vi "TCP server 一对多通讯.vi"() -> ()   [LabVIEW 2015]
uses:
  <vilib>/Analysis/NI_AALBase.lvlib
panel:
  in  "port":u16
  in  "stop":bool
  out "Waveform Graph":dbl[](graph)=[0.0, -0.3446629861261414, 0.6449819459130841, -0.866106479495641, 0.9838729732815561, -0.9870668288033351, 0.878021082565634, -0.6716184455574631, 0.3929433336250866, -0.07396159032953767, -0.25032118712159324, 0.5457579020007043, -0.7825896428232234, 0.9382637669810894, -0.9993074889815294, 0.9621466451128676, -0.8328794880822399, 0.6261206676264622, -0.36311182915767126, 0.0693472019188715, 0.22801633623988113, -0.5027030305125276, 0.7315863059803936, -0.8965016644442846, 0.9854858291916155, -0.9933879258623504, 0.9218598941944436, -0.7787864999433254, 0.5772565526765175, -0.33420418461912077, 0.06886184239247578, 0.1988341088361352, -0.4497566031034409, 0.6669125839906785, -0.83649898302553, 0.9486396514480464, -0.9977828240105574, 0.9827661921181812, -0.9065799590979673, 0.7758761586666735, -0.6002844704019976, 0.3916007514616761, -0.16291497204376829, -0.07225901034618203, 0.30079735532851715, -0.5106798662431301, 0.6915713530529537, -0.8352511156797895, 0.9358828015976429, -0.9901275470744442, 0.997112242978794, -0.9582716672425805, 0.8770879789061665, -0.7587537174921901, 0.6097851702353462, -0.43761202654463116, 0.25016696100073327, -0.055495526672846324, -0.1385971483755034, 0.3248505585398878, -0.49679581216189184, 0.6489412953319964, -0.7768964578302177, 0.8774362101337545, -0.9485108543705275, 0.9892082753602621, -0.9996763045465049, 0.9810137849159348, -0.9351389766759363, 0.8646436335742596, -0.7726404372844417, 0.6626105919055042, -0.5382573376516607, 0.40337001948772405, -0.26170220948298023, 0.11686628573757678, 0.027754141792931248, -0.16907346713967436, 0.3043552605745123, -0.4312462762906236, 0.5477946760053648, -0.6524541934721085, 0.7440761832213633, -0.8218916033501608, 0.8854849932658432, -0.9347624402955282, 0.9699154012496086, -0.9913820727887072, 0.9998078027986025, -0.9960058171624511, 0.9809193135871277, -0.9555857556896089, 0.9211039935631101, -0.878604646809285, 0.8292240161144818, -0.7740816419367104, 0.7142615045606484, -0.6507967584456191, 0.5846578144089939, -0.5167435241375766, 0.4478751807836437, -0.3787930247242358, 0.31015493258496235, -0.24253696800529956, 0.17643548209795307, -0.112270468033949, 0.05038989577020649, 0.008925222046267417, -0.06545525495299609, 0.11903606448288666, -0.16955296546409745, 0.21693467872241692, -0.26114739000849074, 0.30218900684481415, -0.3400836840953238, 0.3748766705541803, -0.40662951278131604, 0.4354156387531364, -0.461316332559608, 0.4844171022317741, -0.5048044356639747, 0.522562934321303, -0.5377728108040681, 0.5505077341839772, -0.5608330061412039, 0.568804051134239, -0.5744652049513441, 0.5778487878598408]
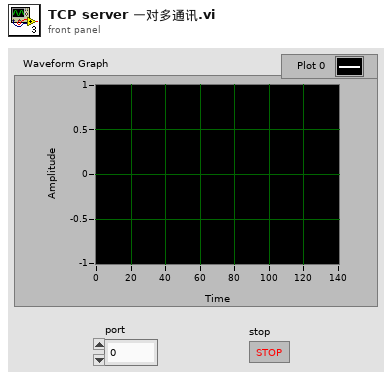
[diagram p1: front panel]
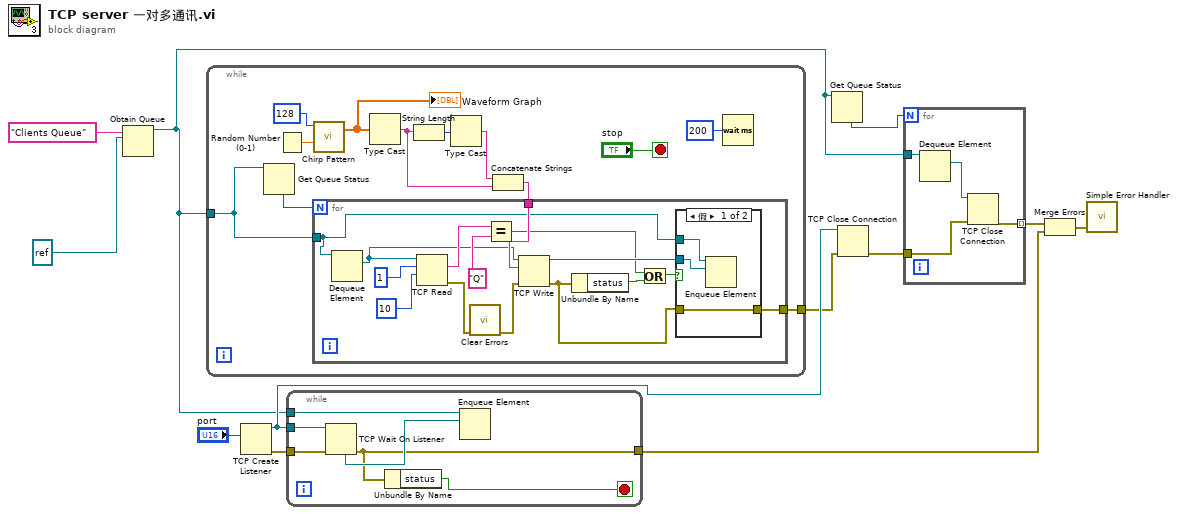
[diagram p0: block diagram]
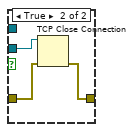
[diagram p2: hidden frame]
diagram:
  n1 = Obtain Queue(name (unnamed)="Clients Queue", element data type=refnum<k5> refnum ("listener ID out")) -> (queue out=w7:refnum<queue>)  [unwired: 3 in, 2 out]
  n2 = while {
    tunnel: w7 -> [w17]
    tunnel: [w15] -> w1
    stop <- "stop" stop-if-true
    n3 = Get Queue Status(queue=w17) -> (# elements in queue=w16:i32)  [unwired: 2 in, 7 out]
    n4 = Random Number (0-1)() -> (number: 0 to 1=w23:dbl)
    n5 = call <vilib>:"Chirp Pattern.vi"("f1"=w23, "samples"=128) -> ("Chirp Pattern"=w14:dbl[])  [unwired: 2 in, 1 out]
    "Waveform Graph" <- w14
    n6 = Type Cast(x=w14) -> (*(type *) &x=w20:string)  [unwired: 1 in]
    n7 = String Length(string=w20) -> (length=w24:i32)
    n8 = Type Cast(x=w24) -> (*(type *) &x=w21:string)  [unwired: 1 in]
    n9 = Concatenate Strings(w21, w20) -> (w19:string)
    n10 = for {
      N: w16 -> [_]
      tunnel: w19 -> [w37]
      tunnel: w17 -> [w29]
      tunnel: [w25] -> w15
      n11 = Dequeue Element(queue=w29) -> (element=w28:refnum<k5>)  [unwired: 2 in, 3 out]
      n12 = TCP Read(connection ID=w28, bytes to read=1, 9:10 ("timeout ms (25000)")) -> (data out=w35:string, error out=w26:errorcluster)  [unwired: 2 in, 1 out]
      n13 = call <vilib>:"Clear Errors.vi"("error in (no error)"=w26) -> ("error out"=w27:errorcluster)  [unwired: 5 in, 1 out]
      n14 = Equal?(x=w35, y="Q") -> (x = y?=w30:bool)
      n15 = TCP Write(connection ID=w28, data in=w37, error in (no error)=w27) -> (connection ID out=w34:refnum<k5>, error out=w32:errorcluster)  [unwired: 1 in, 1 out]
      n16 = Unbundle By Name(w32) -> ("status"=w31:bool)
      n17 = Or(x=w30, y=w31) -> (x .or. y?=w33:bool)
      n18 = case shown="假" w33 {
        tunnel: w32 -> [w42 w45]
        tunnel: w34 -> [w41 w44]
        tunnel: [w42 w43] -> w25
        tunnel: w29 -> [w40 _]
        frame False {
          n19 = Enqueue Element(queue=w40, element=w41) -> ()  [unwired: 2 in, 3 out]
        }
        frame True {
          n20 = TCP Close Connection(connection ID=w44, error in (no error)=w45) -> (error out=w43:errorcluster)  [unwired: 1 in, 1 out]
        }
      }
    }
    n21 = Wait (ms)(milliseconds to wait=u32 200) -> ()  [unwired: 1 out]
  }
  n22 = TCP Create Listener(10:"port") -> (0:w10:errorcluster, 3:w9:refnum<k5>)  [unwired: 4 in, 1 out]
  n23 = while {
    tunnel: w10 -> [w50]
    tunnel: w9 -> [w49]
    tunnel: w7 -> [w47]
    tunnel: [w46] -> w3
    stop <- w51 stop-if-true
    n24 = TCP Wait On Listener(8:w50, 11:w49) -> (0:w46:errorcluster, 4:w48:refnum<k5>)  [unwired: 2 in, 3 out]
    n25 = Unbundle By Name(w46) -> ("status"=w51:bool)
    n26 = Enqueue Element(queue=w47, element=w48) -> ()  [unwired: 2 in, 3 out]
  }
  n27 = Get Queue Status(queue=w7) -> (# elements in queue=w6:i32)  [unwired: 2 in, 7 out]
  n28 = TCP Close Connection(connection ID=w9, error in (no error)=w1) -> (error out=w8:errorcluster)  [unwired: 1 in, 1 out]
  n29 = for {
    N: w6 -> [_]
    tunnel: w8 -> [w55]
    tunnel: w7 -> [w53]
    tunnel: [w54] -> w4 mode=indexing
    n30 = Dequeue Element(queue=w53) -> (element=w52:refnum<k5>)  [unwired: 2 in, 3 out]
    n31 = TCP Close Connection(connection ID=w52, error in (no error)=w55) -> (error out=w54:errorcluster)  [unwired: 1 in, 1 out]
  }
  n32 = Merge Errors(w4, w3) -> (w5:errorcluster)
  n33 = call <vilib>:"Simple Error Handler.vi"("error in (no error)"=w5) -> ()  [unwired: 4 in, 5 out]
